vi "Read WaveformDataArray.vi"(8 "error in (no error)":errorcluster, 11 "NiBase in":refnum<class "NiBase.lvclass">) -> (0 "error out":errorcluster, 2 "WaveformDataArray":waveform(dbl)[](array[waveform]), 3 "NiBase out":refnum<class "NiBase.lvclass">)   [LabVIEW 2014, in "SamplerPlugins.lvlib" / "NiBase.lvclass"]
uses:
  NiBase.lvclass
  NiBase.lvclass/NiBase.ctl
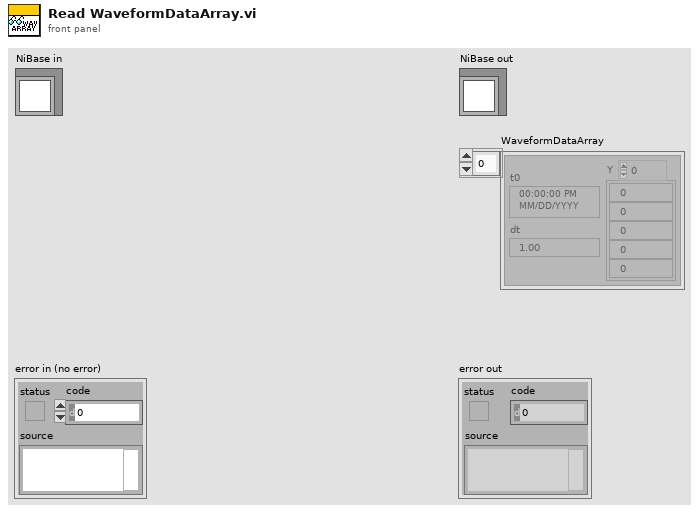
[diagram p1: front panel]
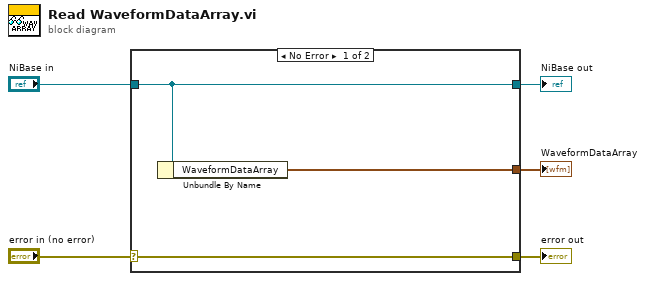
[diagram p0: block diagram]
diagram:
  n1 = case shown="No Error" "error in (no error)" {
    selector: "error in (no error)" -> [w8 w9]
    tunnel: [w8 w9] -> w4
    tunnel: [w7 w10] -> w2
    tunnel: "NiBase in" -> [w7 w10]
    tunnel: [w6 _] -> w1
    frame No Error {
      n2 = Unbundle By Name(w7) -> ("WaveformDataArray"=w6:waveform(dbl)[])
    }
    frame Error {
    }
  }
  "error out" <- w4
  "NiBase out" <- w2
  "WaveformDataArray" <- w1
